vi "Source_ROI Values format specifier-norm values precision.vi"() -> (3 "format (%.3f)":string)   [LabVIEW 2017]
panel:
  # "SUBROUTINE"
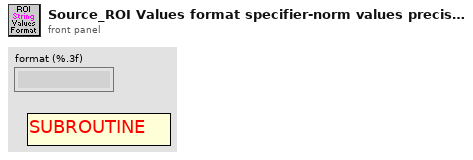
[diagram p1: front panel]
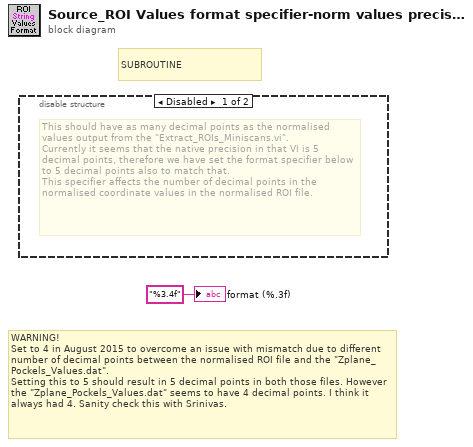
[diagram p0: block diagram]
diagram:
  # "WARNING! \nSet to 4 in August 2015 to overcome an issue with mismatch due to different number of decimal points between the normalised ROI file and the \"Zplane_Pockels_Values.dat\".\nSetting this to 5 should result in 5 decimal points in both those files. However the \"Zplane_Pockels_Values.dat\" seems to have 4 decimal points. I think it always had 4. Sanity check this with Srinivas."
  # "SUBROUTINE"
  n1 = disable-structure shown="Disabled" {
    frame Disabled {
      # "This should have as many decimal points as the normalised values output from the \"Extract_ROIs_Miniscans.vi\".\nCurrently it seems that the native precision in that VI is 5 decimal points, therefore we have set the format specifier below to 5 decimal points also to match that.\nThis specifier affects the number of decimal points in the normalised coordinate values in the normalised ROI file."
    }
    frame Enabled {
    }
  }
  "format (%.3f)" <- "%3.4f" ("format (%.3f)")
